vi "_WriteSubData_TDMS_Control.vi"(8 "error in (no error)":errorcluster, 10 "Sub Data in":T1 {"Control"."motor_ctrl_array"."sensor" format="%#.2f"; "Control"."motor_ctrl_array"."setpoint" format="%#.2f"; "Control"."dac_outputs" format="%#.2f"; "PWR"."motor_array"."motor_name" items=["Motor1", "Motor2", "Motor3", "Motor4", "Motor5", "Motor6"]}, 11 "Refnum in":refnum<k34>) -> (0 "error out":errorcluster, 3 "Refnum out":refnum<k34>)   [LabVIEW 2018]
uses:
  TypeDefsSubsea/Sub Data.ctl
  TypeDefsSubsea/Sub Status.ctl
  Shared/Type Defs/ROV States.ctl
  Shared/Type Defs/SMP.ctl
  Shared/Type Defs/PWR.ctl
  Shared/Type Defs/Motor.ctl
  Shared/Type Defs/MotorNames.ctl
  Shared/Type Defs/SmartCard.ctl
  Shared/Type Defs/Box Names.ctl
  TypeDefsSubsea/Sub Control.ctl
  TypeDefsSubsea/Modos Control.ctl
  TypeDefsSubsea/ROV Outputs.ctl
  TypeDefsSubsea/Motor Control.ctl
  TypeDefsSubsea/Type Defs Subsea.lvlib
  TypeDefsTopside/Type Defs Topside.lvlib
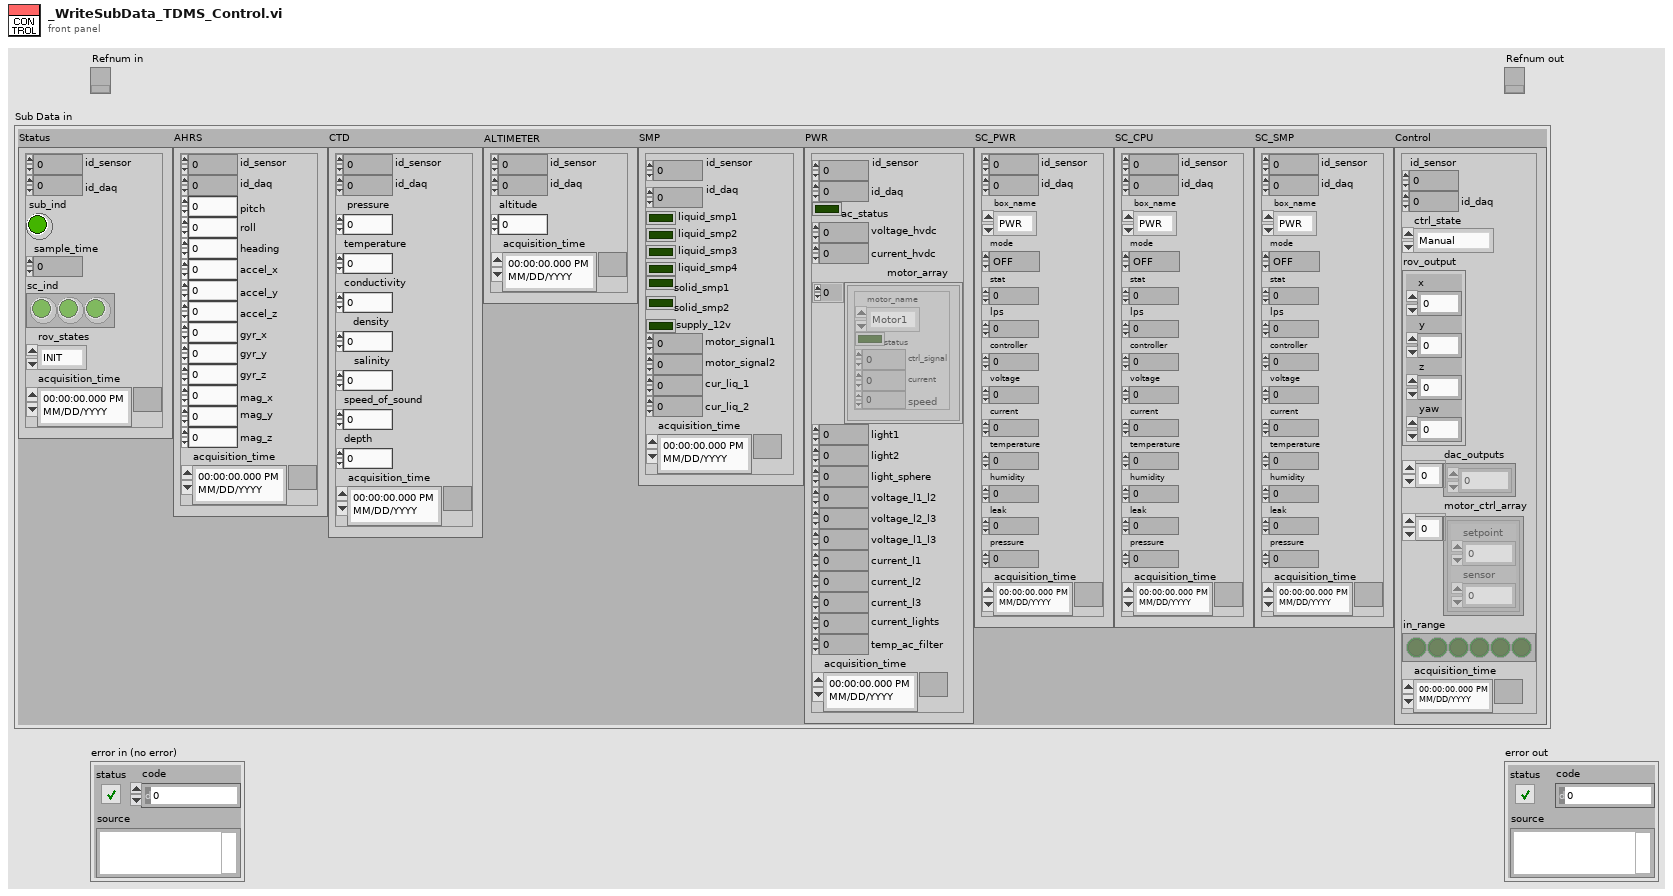
[diagram p1: front panel]
types:
  T1 = typedef "Type Defs Subsea.lvlib/Sub Data.ctl" = cluster{"Status":T2, "AHRS":cluster{"id_sensor":u32, "id_daq":u64, "pitch":dbl, "roll":dbl, "heading":dbl, "accel_x":dbl, "accel_y":dbl, "accel_z":dbl, "gyr_x":dbl, "gyr_y":dbl, "gyr_z":dbl, "mag_x":dbl, "mag_y":dbl, "mag_z":dbl, "acquisition_time":timestamp}, "CTD":cluster{"id_sensor":u32, "id_daq":u64, "pressure":dbl, "temperature":dbl, "conductivity":dbl, "density":dbl, "salinity":dbl, "speed_of_sound":dbl, "depth":dbl, "acquisition_time":timestamp}, "ALTIMETER":cluster{"id_sensor":u32, "id_daq":u64, "altitude":dbl, "acquisition_time":timestamp}, "SMP":T4, "PWR":T5, "SC_PWR":T8, "SC_CPU":T8, "SC_SMP":T8, "Control":T10}
  T2 = typedef "Type Defs Subsea.lvlib/Sub Status.ctl" = cluster{"id_sensor":u32, "id_daq":u32, "sub_ind":bool, "sample_time":i64, "sc_ind":bool[], "rov_states":T3, "acquisition_time":timestamp}
  T3 = typedef "Type Defs Subsea.lvlib/ROV States.ctl" = enum16{"INIT", "IDLE", "TEST", "RUN", "EMERGENCY", "EXIT"}
  T4 = typedef "Type Defs Subsea.lvlib/SMP.ctl" = cluster{"id_sensor":u32, "id_daq":u64, "liquid_smp1":bool, "liquid_smp2":bool, "liquid_smp3":bool, "liquid_smp4":bool, "solid_smp1":bool, "solid_smp2":bool, "supply_12v":bool, "motor_signal1":dbl, "motor_signal2":dbl, "cur_liq_1":dbl, "cur_liq_2":dbl, "acquisition_time":timestamp}
  T5 = typedef "Type Defs Topside.lvlib/PWR.ctl" = cluster{"id_sensor":u32, "id_daq":u64, "ac_status":bool, "voltage_hvdc":dbl, "current_hvdc":dbl, "motor_array":T6[], "light1":dbl, "light2":dbl, "light_sphere":dbl, "voltage_l1_l2":dbl, "voltage_l2_l3":dbl, "voltage_l1_l3":dbl, "current_l1":dbl, "current_l2":dbl, "current_l3":dbl, "current_lights":dbl, "temp_ac_filter":dbl, "acquisition_time":timestamp}
  T6 = typedef "Type Defs Subsea.lvlib/Motor.ctl" = cluster{"motor_name":T7, "status":bool, "ctrl_signal":dbl, "current":dbl, "speed":dbl}
  T7 = typedef "Type Defs Subsea.lvlib/MotorNames.ctl" = u16
  T8 = typedef "Type Defs Subsea.lvlib/SmartCard.ctl" = cluster{"id_sensor":u32, "id_daq":u64, "box_name":T9, "mode":enum16{"OFF", "STANDBY", "TESTING", "RUN", "EMERGENCY"}, "stat":dbl, "lps":dbl, "controller":dbl, "voltage":dbl, "current":dbl, "temperature":dbl, "humidity":dbl, "leak":dbl, "pressure":dbl, "acquisition_time":timestamp}
  T9 = typedef "Type Defs Subsea.lvlib/Box Names.ctl" = enum16{"PWR", "CPU", "SMP"}
  T10 = typedef "Type Defs Subsea.lvlib/Sub Control.ctl" = cluster{"id_sensor":u32, "id_daq":u64, "ctrl_state":T11, "rov_output":T12, "dac_outputs":dbl[], "motor_ctrl_array":T13[], "in_range":bool[], "acquisition_time":timestamp}
  T11 = typedef "Type Defs Subsea.lvlib/Modos Control.ctl" = enum16{"Manual", "Profundidad", "Altitud", "Rumbo", "P+R"}
  T12 = typedef "Type Defs Subsea.lvlib/ROV Outputs.ctl" = cluster{"x":dbl, "y":dbl, "z":dbl, "yaw":dbl}
  T13 = typedef "Type Defs Subsea.lvlib/Motor Control.ctl" = cluster{"setpoint":dbl, "sensor":dbl}
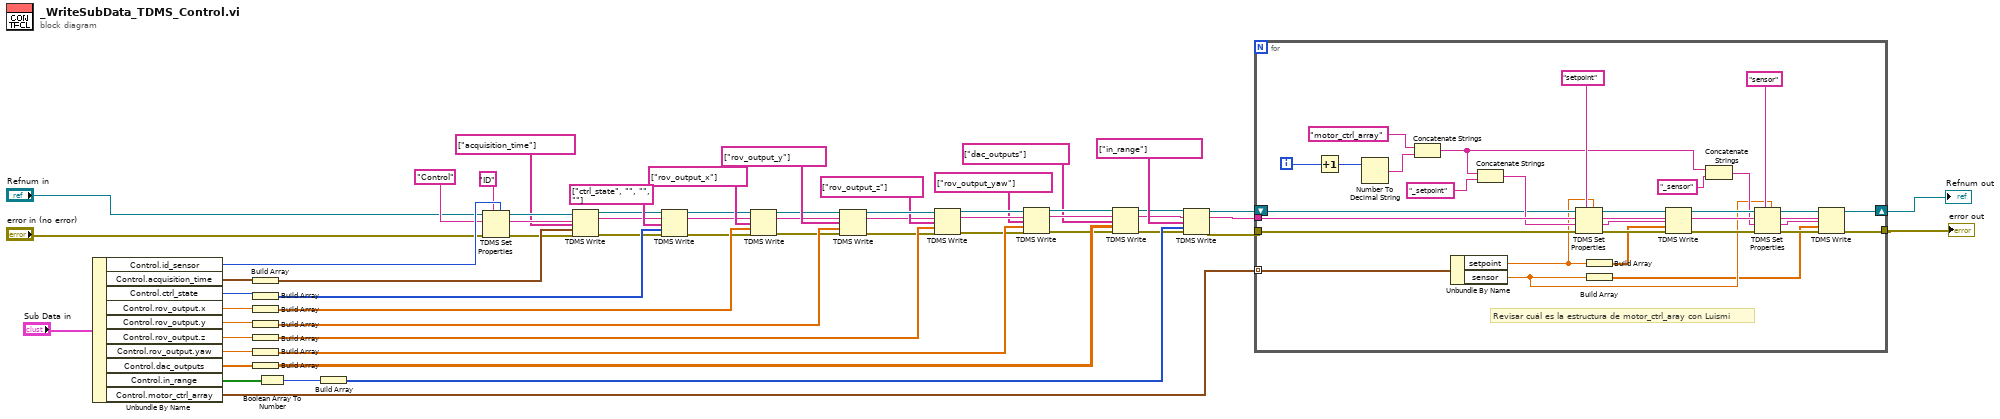
[diagram p0: block diagram]
diagram:
  n1 = Unbundle By Name("Sub Data in") -> ("Control.id_sensor"=w51:u32, "Control.acquisition_time"=w52:timestamp, "Control.ctrl_state"=w53:T11, "Control.rov_output.x"=w10:dbl, "Control.rov_output.y"=w9:dbl, "Control.rov_output.z"=w8:dbl, "Control.rov_output.yaw"=w7:dbl, "Control.dac_outputs"=w11:dbl[], "Control.in_range"=w1:bool[], "Control.motor_ctrl_array"=w3:T13[])
  n2 = Build Array(w52) -> (w54:timestamp[])
  n3 = Build Array(w53) -> (w55:T11[])
  n4 = Build Array(w10) -> (w56:dbl[])
  n5 = Build Array(w9) -> (w57:dbl[])
  n6 = Build Array(w8) -> (w58:dbl[])
  n7 = Build Array(w7) -> (w59:dbl[])
  n8 = Build Array(w11) -> (w60:dbl[][])
  n9 = Boolean Array To Number(Boolean array=w1) -> (number=w2:u32)
  n10 = Build Array(w2) -> (w61:u32[])
  n11 = TDMS Set Properties(5:w51, 7:"ID" ("property names"), 8:"error in (no error)", 10:"Control" ("group name in (Untitled)"), 11:"Refnum in") -> (0:w30:errorcluster, 2:w29:string, 3:w27:refnum<k34>)  [unwired: 1 in, 1 out]
  n12 = TDMS Write(0:w27, 5:w29, 7:string[] ["acquisition_time"] ("channel name(s) in (Untitled)"), 9:w54, 11:w30) -> (4:w23:refnum<k34>, 6:w22:string, 15:w24:errorcluster)  [unwired: 1 in, 1 out]
  n13 = TDMS Write(0:w23, 5:w22, 7:string[] ["ctrl_state", "", "", ""] ("channel name(s) in (Untitled)"), 9:w55, 11:w24) -> (4:w35:refnum<k34>, 6:w34:string, 15:w36:errorcluster)  [unwired: 1 in, 1 out]
  n14 = TDMS Write(0:w35, 5:w34, 7:string[] ["rov_output_x"] ("channel name(s) in (Untitled)"), 9:w56, 11:w36) -> (4:w32:refnum<k34>, 6:w31:string, 15:w33:errorcluster)  [unwired: 1 in, 1 out]
  n15 = TDMS Write(0:w32, 5:w31, 7:string[] ["rov_output_y"] ("channel name(s) in (Untitled)"), 9:w57, 11:w33) -> (4:w16:refnum<k34>, 6:w14:string, 15:w17:errorcluster)  [unwired: 1 in, 1 out]
  n16 = TDMS Write(0:w16, 5:w14, 7:string[] ["rov_output_z"] ("channel name(s) in (Untitled)"), 9:w58, 11:w17) -> (4:w42:refnum<k34>, 6:w43:string, 15:w41:errorcluster)  [unwired: 1 in, 1 out]
  n17 = TDMS Write(0:w42, 5:w43, 7:string[] ["rov_output_yaw"] ("channel name(s) in (Untitled)"), 9:w59, 11:w41) -> (4:w45:refnum<k34>, 6:w46:string, 15:w44:errorcluster)  [unwired: 1 in, 1 out]
  n18 = TDMS Write(0:w45, 5:w46, 7:string[] ["dac_outputs"] ("channel name(s) in (Untitled)"), 9:w60, 11:w44) -> (4:w47:refnum<k34>, 6:w49:string, 15:w48:errorcluster)  [unwired: 1 in, 1 out]
  n19 = TDMS Write(0:w47, 5:w49, 7:string[] ["in_range"] ("channel name(s) in (Untitled)"), 9:w61, 11:w48) -> (4:w6:refnum<k34>, 6:w5:string, 15:w4:errorcluster)  [unwired: 1 in, 1 out]
  n20 = for {
    tunnel: w3 -> [w87] mode=indexing
    tunnel: w4 -> [w82]
    tunnel: w5 -> [w81]
    shift-right: [w69] -> w12
    shift-left: w6 -> [w71]
    tunnel: [w70] -> w13
    i -> [w85]
    # "Revisar cuál es la estructura de motor_ctrl_aray con Luismi"
    n21 = Increment(x=w85) -> (x+1=w86:i32)
    n22 = Number To Decimal String(number=w86) -> (decimal integer string=w83:string)  [unwired: 1 in]
    n23 = Concatenate Strings("motor_ctrl_array" ("string"), w83) -> (w72:string)
    n24 = Unbundle By Name(w87) -> ("setpoint"=w67:dbl, "sensor"=w64:dbl)
    n25 = Concatenate Strings(w72, "_setpoint" ("string")) -> (w75:string)
    n26 = TDMS Set Properties(5:w67, 7:"setpoint" ("property names"), 8:w82, 9:w75, 10:w81, 11:w71) -> (0:w91:errorcluster, 1:w68:string, 2:w78:string, 3:w77:refnum<k34>)
    n27 = Build Array(w67) -> (w66:dbl[])
    n28 = Build Array(w64) -> (w62:dbl[])
    n29 = TDMS Write(0:w77, 5:w78, 7:w68, 9:w66, 11:w91) -> (4:w76:refnum<k34>, 6:w92:string, 15:w80:errorcluster)  [unwired: 1 in, 1 out]
    n30 = Concatenate Strings(w72, "_sensor" ("string")) -> (w73:string)
    n31 = TDMS Set Properties(5:w64, 7:"sensor" ("property names"), 8:w80, 9:w73, 10:w92, 11:w76) -> (0:w88:errorcluster, 1:w63:string, 2:w90:string, 3:w89:refnum<k34>)
    n32 = TDMS Write(0:w89, 5:w90, 7:w63, 9:w62, 11:w88) -> (4:w69:refnum<k34>, 15:w70:errorcluster)  [unwired: 1 in, 2 out]
  }
  "error out" <- w13
  "Refnum out" <- w12
